vi "Set camera exposure.vi"(0 "Camera reference in":refnum<k24>, 2 "Exposure time (ms)":dbl, 5 "Error In":errorcluster) -> (14 "Camera reference out":refnum<k24>, 19 "Error Out":errorcluster)   [LabVIEW 2017]
uses:
  C:/Program Files/National Instruments/LabVIEW 2017/instr.lib/IDS/ueye.NET/uEyeDotNet.dll
panel:
  out "Actual exposure time (ms)":dbl
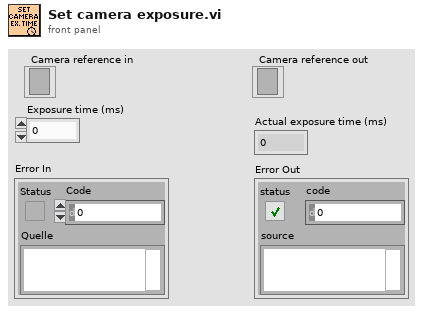
[diagram p1: front panel]
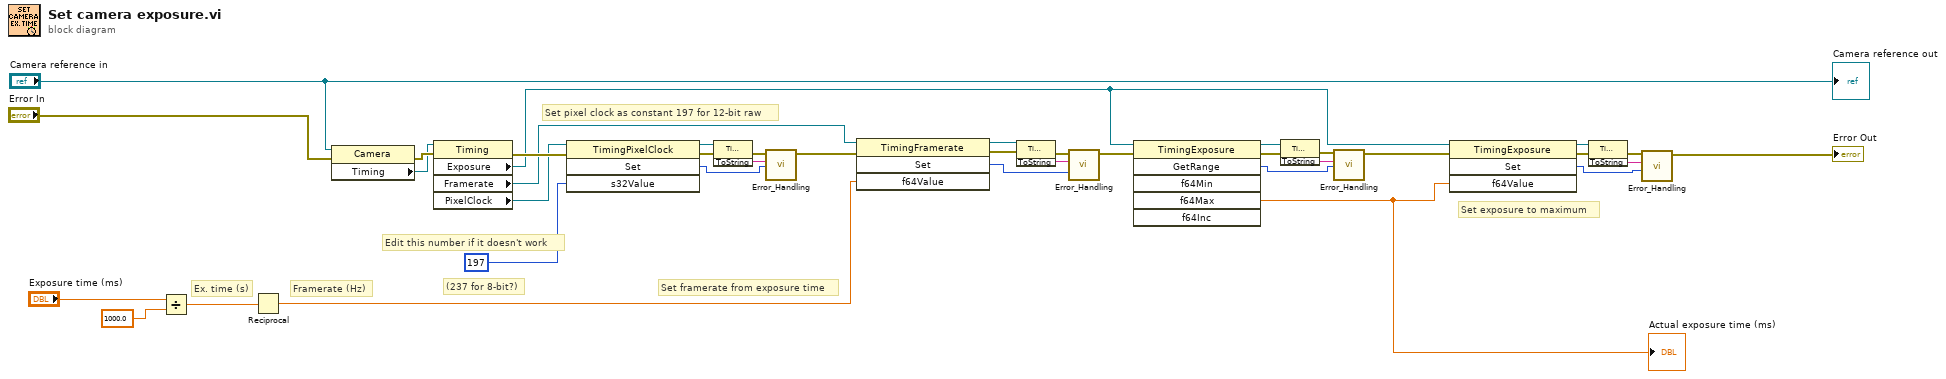
[diagram p0: block diagram]
diagram:
  # "Set exposure to maximum"
  # "(237 for 8-bit?)"
  # "Set framerate from exposure time"
  # "Edit this number if it doesn't work"
  # "Set pixel clock as constant 197 for 12-bit raw"
  # "Framerate (Hz)"
  # "Ex. time (s)"
  n1 = Divide(x="Exposure time (ms)", y=1000.0) -> (x/y=w37:dbl)
  n2 = Reciprocal(x=w37) -> (1/x=w22:dbl)
  n3 = property class="Camera"(reference="Camera reference in", error in="Error In") -> (error out=w36:errorcluster, "Timing"=w35:refnum<k24>)  [unwired: 1 out]
  n4 = property class="Timing"(reference=w35, error in=w36) -> (error out=w29:errorcluster, "Exposure"=w16:refnum<k24>, "Framerate"=w20:refnum<k24>, "PixelClock"=w21:refnum<k24>)  [unwired: 1 out]
  n5 = invoke class="TimingPixelClock" method="Set"(reference=w21, error in=w29, "s32Value"=197) -> (reference out=w25:refnum<k24>, error out=w26:errorcluster, "Set"=w24:i32)  [unwired: 1 in, 1 out]
  n6 = invoke class="TimingPixelClock" method="ToString"(reference=w25, error in=w26) -> (error out=w28:errorcluster, "ToString"=w17:string)  [unwired: 1 in, 1 out]
  n7 = call <instrlib>:"Error_Handling.vi"("Error Code"=w24, "Error String"=w17, "Error In"=w28) -> ("Error Out"=w27:errorcluster)  [unwired: 8 in]
  n8 = invoke on="Methodenknoten" class="TimingFramerate" method="Set"(reference=w20, error in=w27, "f64Value"=w22) -> (reference out=w33:refnum<k24>, error out=w32:errorcluster, "Set"=w30:i32)  [unwired: 1 in, 1 out]
  n9 = invoke class="TimingFramerate" method="ToString"(reference=w33, error in=w32) -> (error out=w31:errorcluster, "ToString"=w18:string)  [unwired: 1 in, 1 out]
  n10 = call <instrlib>:"Error_Handling.vi"("Error Code"=w30, "Error String"=w18, "Error In"=w31) -> ("Error Out"=w19:errorcluster)  [unwired: 8 in]
  n11 = invoke class="TimingExposure" method="GetRange"(reference=w16, error in=w19) -> (reference out=w9:refnum<k24>, error out=w10:errorcluster, "GetRange"=w11:i32, "f64Max"=w14:dbl)  [unwired: 4 in, 2 out]
  "Actual exposure time (ms)" <- w14
  n12 = invoke class="TimingExposure" method="ToString"(reference=w9, error in=w10) -> (error out=w13:errorcluster, "ToString"=w12:string)  [unwired: 1 in, 1 out]
  n13 = call <instrlib>:"Error_Handling.vi"("Error Code"=w11, "Error String"=w12, "Error In"=w13) -> ("Error Out"=w8:errorcluster)  [unwired: 8 in]
  n14 = invoke class="TimingExposure" method="Set"(reference=w16, error in=w8, "f64Value"=w14) -> (reference out=w2:refnum<k24>, error out=w3:errorcluster, "Set"=w4:i32)  [unwired: 1 in, 1 out]
  n15 = invoke class="TimingExposure" method="ToString"(reference=w2, error in=w3) -> (error out=w6:errorcluster, "ToString"=w5:string)  [unwired: 1 in, 1 out]
  n16 = call <instrlib>:"Error_Handling.vi"("Error Code"=w4, "Error String"=w5, "Error In"=w6) -> ("Error Out"=→"Error Out":errorcluster)  [unwired: 8 in]
  "Camera reference out" <- "Camera reference in"
